vi "SPD.Get DT Histo File.vi"(6 "DT folder":bool, 8 "Error In":errorcluster, 9 "DT":dbl, 10 "Insens":dbl, 11 "SPD.Stand Ctrl in":T1={"spdDeviceSession"={"spdRef"=0, "connected"=FALSE, "spdName"="", "specification"={"diod case"=enum."default", "type"=enum."Unknown", "frequency"=enum."Unknown"}, "hidSPD.Controller"={"TSet"=0.0, "HV_bias"=0.0, "DDS_stb_code"=0}, "hidSPD.Sturtup Values"={"TSet"=0.0, "HV_bias"=0.0, "DDS_stb_code"=0}}, "DevBSession"={"DevBRef"="", "connected"=FALSE}, "FreqCSession"={"FreqCRef"="", "timeout"=0.0, "Gate"=0.0, "connected"=FALSE}, "8164BSession"={"Connection ID"=refnum, "Connected"=FALSE, "Info"="", "Slots Info"=[]}, "LeCroySession"={"LeCroySession"="", "connected"=FALSE}, "Events"={"DCRTest"=refnum, "Stop"=refnum}, "configFile"={"configFile ref"=refnum, "configFile path"=path "", "equipmentFile ref"=refnum}, "SPD.Meas Grid"={"DateTime"="", "DT"=[], "Insensitivity"=[], "Temprature"=[], "Stb_code"=[], "HV_Bias"=[]}, "SPD.Queues"={"state queue"=refnum}, "Console"=refnum} {"spdDeviceSession"."hidSPD.Sturtup Values"."HV_bias" format="%#_6p, V"; "spdDeviceSession"."hidSPD.Sturtup Values"."TSet" format="%#_6p, DegC"; "spdDeviceSession"."hidSPD.Controller"."HV_bias" format="%#_6p, V"; "spdDeviceSession"."hidSPD.Controller"."TSet" format="%#_6p, DegC"}) -> (0 "Error Out":errorcluster, 2 "DT Results path":path, 3 "SPD.Stand Ctrl out":T1={"spdDeviceSession"={"spdRef"=0, "connected"=FALSE, "spdName"="", "specification"={"diod case"=enum."default", "type"=enum."Unknown", "frequency"=enum."Unknown"}, "hidSPD.Controller"={"TSet"=0.0, "HV_bias"=0.0, "DDS_stb_code"=0}, "hidSPD.Sturtup Values"={"TSet"=0.0, "HV_bias"=0.0, "DDS_stb_code"=0}}, "DevBSession"={"DevBRef"="", "connected"=FALSE}, "FreqCSession"={"FreqCRef"="", "timeout"=0.0, "Gate"=0.0, "connected"=FALSE}, "8164BSession"={"Connection ID"=refnum, "Connected"=FALSE, "Info"="", "Slots Info"=[]}, "LeCroySession"={"LeCroySession"="", "connected"=FALSE}, "Events"={"DCRTest"=refnum, "Stop"=refnum}, "configFile"={"configFile ref"=refnum, "configFile path"=path "", "equipmentFile ref"=refnum}, "SPD.Meas Grid"={"DateTime"="", "DT"=[], "Insensitivity"=[], "Temprature"=[], "Stb_code"=[], "HV_Bias"=[]}, "SPD.Queues"={"state queue"=refnum}, "Console"=refnum} {"spdDeviceSession"."hidSPD.Sturtup Values"."HV_bias" format="%#_6p, V"; "spdDeviceSession"."hidSPD.Sturtup Values"."TSet" format="%#_6p, DegC"; "spdDeviceSession"."hidSPD.Controller"."HV_bias" format="%#_6p, V"; "spdDeviceSession"."hidSPD.Controller"."TSet" format="%#_6p, DegC"})   [LabVIEW 2018]
uses:
  typedefs/SPD.Stand Ctrl.ctl
  Instruments/SPD HID Interface/hidSPDLibForLabView/LibVIs/hidSPD Controls/hidSPD Device Session.ctl
  Instruments/SPD HID Interface/hidSPDLibForLabView/LibVIs/hidSPD Controls/hidSPD.SPD specification.ctl
  Instruments/SPD HID Interface/hidSPDLibForLabView/LibVIs/hidSPD Controls/hidSPD SPD Diod Case.ctl
  Instruments/SPD HID Interface/hidSPDLibForLabView/LibVIs/hidSPD Controls/hidSPD SPD Type.ctl
  Instruments/SPD HID Interface/hidSPDLibForLabView/LibVIs/hidSPD Controls/hidSPD.STB Frequency.ctl
  Instruments/SPD HID Interface/hidSPDLibForLabView/LibVIs/hidSPD Controls/hidSPD Controller.ctl
  Instruments/KC705 DevBoard/typedefs/DevB.Session.ctl
  Instruments/KeySight 53230A/typedefs/FreqC.Session.ctl
  Instruments/KeySight 8164B/KeySight 8164B LAN InstrLib/typedefs/KeySight 8164B control.ctl
  Instruments/LeCroy SDA830/typedefs/LeCroy.Session.ctl
  typedefs/SPD.Events.ctl
  ConfigFile/SPD.Config File ctrl.ctl
  <vilib>/Utility/config.llb/Config Data RefNum.ctl
  typedefs/SPD.Meas Grid.ctl
  typedefs/SPD.Queues.ctl
  typedefs/SPD.Stand state.ctl
  <vilib>/Utility/sysdir.llb/System Directory Type.ctl
  Instruments/KeySight 8164B/KeySight 8164B LAN InstrLib.lvlib
  <vilib>/Utility/config.llb/NI_LVConfig.lvlib
  Instruments/SPD HID Interface/hidSPDLibForLabView/hidSPDLibForLabView.lvlib
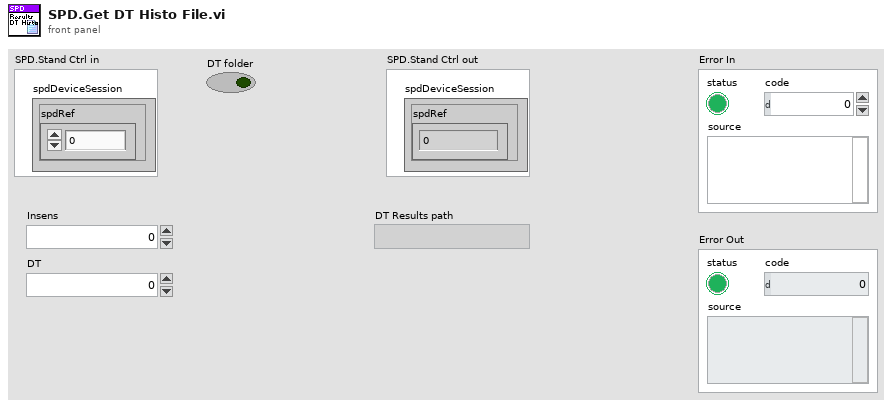
[diagram p1: front panel]
types:
  T1 = typedef "SPD.Stand Ctrl.ctl" = cluster{"spdDeviceSession":T2, "DevBSession":T8, "FreqCSession":T9, "8164BSession":T10, "LeCroySession":T11, "Events":T12, "configFile":T13, "SPD.Meas Grid":T15, "SPD.Queues":T16, "Console":refnum<vi>}
  T2 = typedef "hidSPDLibForLabView.lvlib/hidSPD Device Session.ctl" = cluster{"spdRef":u64, "connected":bool, "spdName":string, "specification":T3, "hidSPD.Controller":T7, "hidSPD.Sturtup Values":T7}
  T3 = typedef "hidSPDLibForLabView.lvlib/hidSPD.SPD specification.ctl" = cluster{"diod case":T4, "type":T5, "frequency":T6}
  T4 = typedef "hidSPDLibForLabView.lvlib/hidSPD SPD Diod Case.ctl" = enum16{"Unknown", "default", "butterfly"}
  T5 = typedef "hidSPDLibForLabView.lvlib/hidSPD SPD Type.ctl" = enum16{"Unknown", "Free Run", "Gate"}
  T6 = typedef "hidSPDLibForLabView.lvlib/hidSPD.STB Frequency.ctl" = enum16{"Unknown", "312", "1250"}
  T7 = typedef "hidSPDLibForLabView.lvlib/hidSPD Controller.ctl" = cluster{"TSet":sgl, "HV_bias":sgl, "DDS_stb_code":u16}
  T8 = typedef "DevB.Session.ctl" = cluster{"DevBRef":refnum<visa-resource-name>, "connected":bool}
  T9 = typedef "FreqC.Session.ctl" = cluster{"FreqCRef":refnum<visa-resource-name>, "timeout":dbl, "Gate":dbl, "connected":bool}
  T10 = typedef "KeySight 8164B LAN InstrLib.lvlib/KeySight 8164B control.ctl" = cluster{"Connection ID":refnum<k5>, "Connected":bool, "Info":string, "Slots Info":string[]}
  T11 = typedef "LeCroy.Session.ctl" = cluster{"LeCroySession":refnum<visa-resource-name>, "connected":bool}
  T12 = typedef "SPD.Events.ctl" = cluster{"DCRTest":refnum<user-event>, "Stop":refnum<user-event>}
  T13 = typedef "SPD.Config File ctrl.ctl" = cluster{"configFile ref":T14, "configFile path":path, "equipmentFile ref":T14}
  T14 = typedef "NI_LVConfig.lvlib/Config Data RefNum.ctl" = refnum<k1>
  T15 = typedef "SPD.Meas Grid.ctl" = cluster{"DateTime":string, "DT":dbl[], "Insensitivity":dbl[], "Temprature":dbl[], "Stb_code":dbl[], "HV_Bias":dbl[][][][]}
  T16 = typedef "SPD.Queues.ctl" = cluster{"state queue":refnum<queue>}
  T17 = typedef "System Directory Type.ctl" = i32
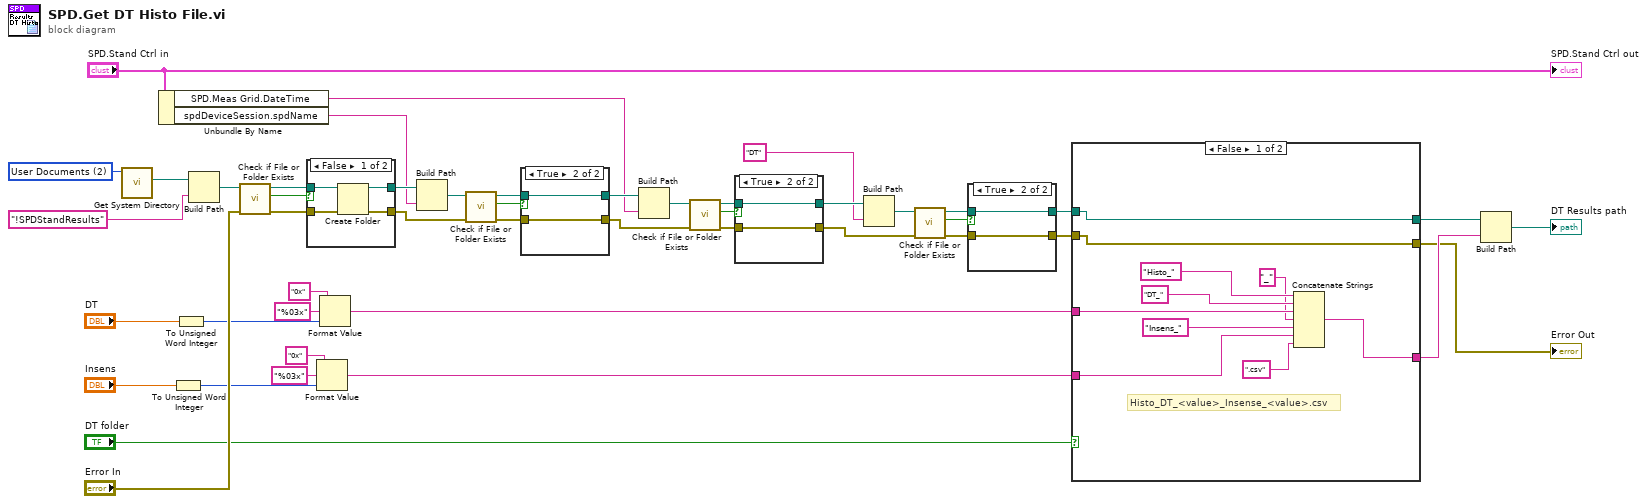
[diagram p0: block diagram]
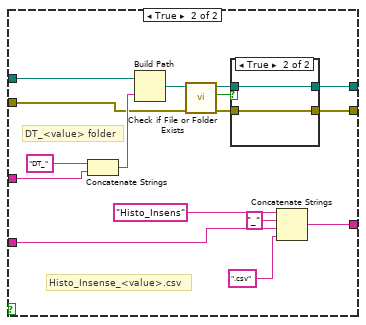
[diagram p2: hidden frame]
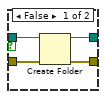
[diagram p3: hidden frame]
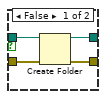
[diagram p4: hidden frame]
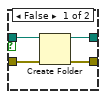
[diagram p5: hidden frame]
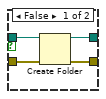
[diagram p6: hidden frame]
diagram:
  w47 = T17 2 items=["User Home"=0, "User Desktop"=1, "User Documents"=2, "User Application Data"=3, "User Preferences"=4, "User Temporary"=5, "Public Documents"=6, "Public Application Data"=7, "Public Preferences"=8, "Public Cache"=13, "System Core Libraries"=9, "System Installed Libraries"=10, "Application Files"=11, "Boot Volume Root"=12] ("system directory type")
  n1 = call <vilib>:"Get System Directory.vi"("system directory type"=w47) -> ("system directory"=w46:path)  [unwired: 10 in]
  n2 = Unbundle By Name("SPD.Stand Ctrl in") -> ("SPD.Meas Grid.DateTime"=w30:string, "spdDeviceSession.spdName"=w37:string)
  n3 = To Unsigned Word Integer(number="Insens") -> (unsigned 16bit integer=w23:u16)
  n4 = To Unsigned Word Integer(number="DT") -> (unsigned 16bit integer=w16:u16)
  n5 = Build Path(base path=w46, name or relative path="!SPDStandResults") -> (appended path=w44:path)
  n6 = call <vilib>:"Check if File or Folder Exists.vi"("error in (no error)"="Error In", "path"=w44) -> ("error out"=w40:errorcluster, "file or folder exists?"=w42:bool, "dup path"=w41:path)  [unwired: 7 in]
  n7 = case shown="False" w42 {
    tunnel: w41 -> [w51 w53]
    tunnel: w40 -> [w50 w52]
    tunnel: [w49 w53] -> w39
    tunnel: [w48 w52] -> w35
    frame False {
      n8 = Create Folder(path (use dialog)=w51, error in=w50) -> (created path=w49:path, error out=w48:errorcluster)  [unwired: 1 in, 1 out]
    }
    frame True {
    }
  }
  n9 = Format Value(string ("")="0x", format string="%03x", value (0)=w23) -> (output string=w6:string)
  n10 = Format Value(string ("")="0x", format string="%03x", value (0)=w16) -> (output string=w18:string)
  n11 = Build Path(base path=w39, name or relative path=w37) -> (appended path=w36:path)
  n12 = call <vilib>:"Check if File or Folder Exists.vi"("error in (no error)"=w35, "path"=w36) -> ("error out"=w32:errorcluster, "file or folder exists?"=w33:bool, "dup path"=w34:path)  [unwired: 7 in]
  n13 = case shown="True" w33 {
    tunnel: w34 -> [w57 w59]
    tunnel: w32 -> [w56 w58]
    tunnel: [w55 w59] -> w31
    tunnel: [w54 w58] -> w28
    frame False {
      n14 = Create Folder(path (use dialog)=w57, error in=w56) -> (created path=w55:path, error out=w54:errorcluster)  [unwired: 1 in, 1 out]
    }
    frame True {
    }
  }
  n15 = Build Path(base path=w31, name or relative path=w30) -> (appended path=w29:path)
  n16 = call <vilib>:"Check if File or Folder Exists.vi"("error in (no error)"=w28, "path"=w29) -> ("error out"=w25:errorcluster, "file or folder exists?"=w26:bool, "dup path"=w27:path)  [unwired: 7 in]
  n17 = case shown="True" w26 {
    tunnel: w27 -> [w63 w65]
    tunnel: w25 -> [w62 w64]
    tunnel: [w61 w65] -> w11
    tunnel: [w60 w64] -> w10
    frame False {
      n18 = Create Folder(path (use dialog)=w63, error in=w62) -> (created path=w61:path, error out=w60:errorcluster)  [unwired: 1 in, 1 out]
    }
    frame True {
    }
  }
  n19 = Build Path(base path=w11, name or relative path="DT") -> (appended path=w12:path)
  n20 = call <vilib>:"Check if File or Folder Exists.vi"("error in (no error)"=w10, "path"=w12) -> ("error out"=w15:errorcluster, "file or folder exists?"=w14:bool, "dup path"=w13:path)  [unwired: 7 in]
  n21 = case shown="True" w14 {
    tunnel: w13 -> [w69 w71]
    tunnel: w15 -> [w68 w70]
    tunnel: [w67 w71] -> w7
    tunnel: [w66 w70] -> w8
    frame False {
      n22 = Create Folder(path (use dialog)=w69, error in=w68) -> (created path=w67:path, error out=w66:errorcluster)  [unwired: 1 in, 1 out]
    }
    frame True {
    }
  }
  n23 = case shown="False" "DT folder" {
    tunnel: w18 -> [w77 w91]
    tunnel: w8 -> [w73 w90]
    tunnel: w7 -> [w72 w89]
    tunnel: w6 -> [w76 w85]
    tunnel: [w72 w84] -> w5
    tunnel: [w74 w83] -> w4
    tunnel: [w73 w82] -> w3
    frame False {
      # "Histo_DT_<value>_Insense_<value>.csv"
      n24 = Concatenate Strings("Histo_" ("Name"), "DT_" ("string"), w77, "_" ("string"), "Insens_" ("Name"), w76, ".csv" ("string")) -> (w74:string)
    }
    frame True {
      # "DT_<value> folder"
      # "Histo_Insense_<value>.csv"
      n25 = Concatenate Strings("DT_" ("string"), w91) -> (w92:string)
      n26 = Build Path(base path=w89, name or relative path=w92) -> (appended path=w94:path)
      n27 = call <vilib>:"Check if File or Folder Exists.vi"("error in (no error)"=w90, "path"=w94) -> ("error out"=w97:errorcluster, "file or folder exists?"=w96:bool, "dup path"=w95:path)  [unwired: 7 in]
      n28 = case shown="True" w96 {
        tunnel: w95 -> [w101 w103]
        tunnel: w97 -> [w100 w102]
        tunnel: [w99 w103] -> w84
        tunnel: [w98 w102] -> w82
        frame False {
          n29 = Create Folder(path (use dialog)=w101, error in=w100) -> (created path=w99:path, error out=w98:errorcluster)  [unwired: 1 in, 1 out]
        }
        frame True {
        }
      }
      n30 = Concatenate Strings("Histo_Insens" ("Name"), "_" ("string"), w85, ".csv" ("string")) -> (w83:string)
    }
  }
  "Error Out" <- w3
  n31 = Build Path(base path=w5, name or relative path=w4) -> (appended path=→"DT Results path":path)
  "SPD.Stand Ctrl out" <- "SPD.Stand Ctrl in"
